vi "Node - Update Channel Values.vi"(8 "error in (no error)":errorcluster, 10 "Channels In":dbl[](array[numeric]), 11 "Node Data In":T1) -> (0 "error out":errorcluster, 3 "Node Data Out":T1)   [LabVIEW 2016, in "PXImc Router.lvlib"]
uses:
  PXImc Router.lvlib
  Controls/Node Data.ctl
  <vilib>/NI Veristand/VeriStand Data/Byte Buffer/Byte Buffer.lvclass
  Controls/Node/Node - PXImc Parameters.ctl
  Controls/Node/Transfer Data.ctl
  Controls/Node/Node Ch Properties.ctl
  Controls/Data Type.ctl
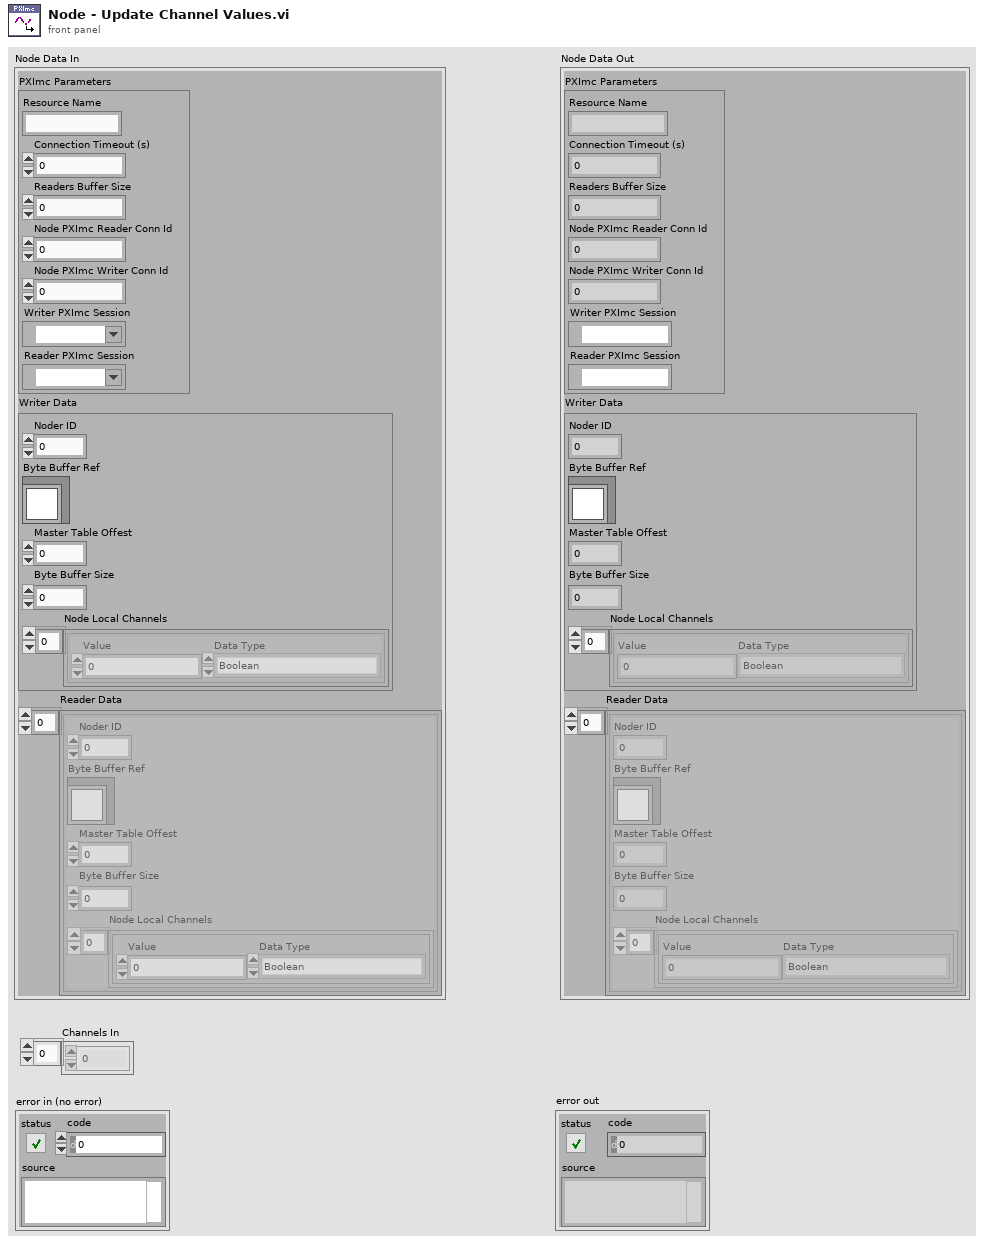
[diagram p1: front panel]
types:
  T1 = typedef "PXImc Router.lvlib/Node Data.ctl" = cluster{"PXImc Parameters":T2, "Writer Data":T3, "Reader Data":T3[]}
  T2 = typedef "PXImc Router.lvlib/Node - PXImc Parameters.ctl" = cluster{"Resource Name":string, "Connection Timeout (s)":dbl, "Readers Buffer Size":u32, "Node PXImc Reader Conn Id":u16, "Node PXImc Writer Conn Id":u16, "Writer PXImc Session":refnum<k21>, "Reader PXImc Session":refnum<k21>}
  T3 = typedef "PXImc Router.lvlib/Transfer Data.ctl" = cluster{"Noder ID":u32, "Byte Buffer Ref":refnum<class "Byte Buffer.lvclass">, "Master Table Offest":u32, "Byte Buffer Size":u32, "Node Local Channels":T4[]}
  T4 = typedef "PXImc Router.lvlib/Node Ch Properties.ctl" = cluster{"Value":dbl, "Data Type":T5}
  T5 = typedef "PXImc Router.lvlib/Data Type.ctl" = enum16{"Boolean", "SGL", "DBL", "I8", "I16", "I32", "I64", "U8", "U16", "U32", "U64"}
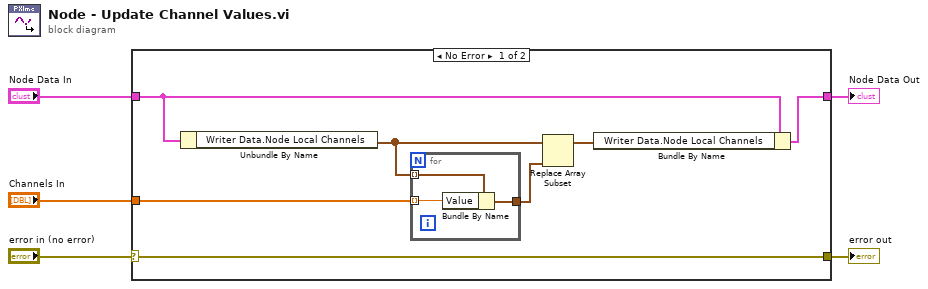
[diagram p0: block diagram]
diagram:
  n1 = case shown="No Error" "error in (no error)" {
    selector: "error in (no error)" -> [w6 w16]
    tunnel: "Node Data In" -> [w12 w17]
    tunnel: "Channels In" -> [w9 _]
    tunnel: [w7 w17] -> w2
    tunnel: [w6 w16] -> w1
    frame No Error {
      n2 = Unbundle By Name(w12) -> ("Writer Data.Node Local Channels"=w8:T4[])
      n3 = for {
        tunnel: [w15] -> w10
        tunnel: w9 -> [w14] mode=indexing
        tunnel: w8 -> [w13] mode=indexing
        n4 = Bundle By Name(cluster=w13, "Value"=w14) -> (w15:T4)
      }
      n5 = Replace Array Subset(array=w8, new element=w10) -> (w11:T4[])  [unwired: 1 in]
      n6 = Bundle By Name(cluster=w12, "Writer Data.Node Local Channels"=w11) -> (w7:T1)
    }
    frame Error {
    }
  }
  "Node Data Out" <- w2
  "error out" <- w1
